vi "Read and Log Data.vi"(6 "Test No.":i32, 7 "Voltage Threshold":dbl=100.0, 8 "error in":errorcluster, 9 "Only Temperature":bool, 10 "Data":waveform(dbl)[](array[waveform]), 11 "tdms file":refnum<k34>) -> (0 "error out":errorcluster, 2 "Voltage Less Than Threshold":bool, 3 "tdms file out":refnum<k34>)   [LabVIEW 2015]
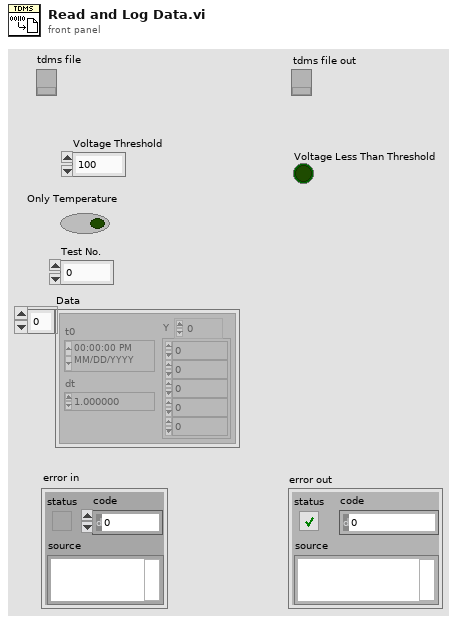
[diagram p1: front panel]
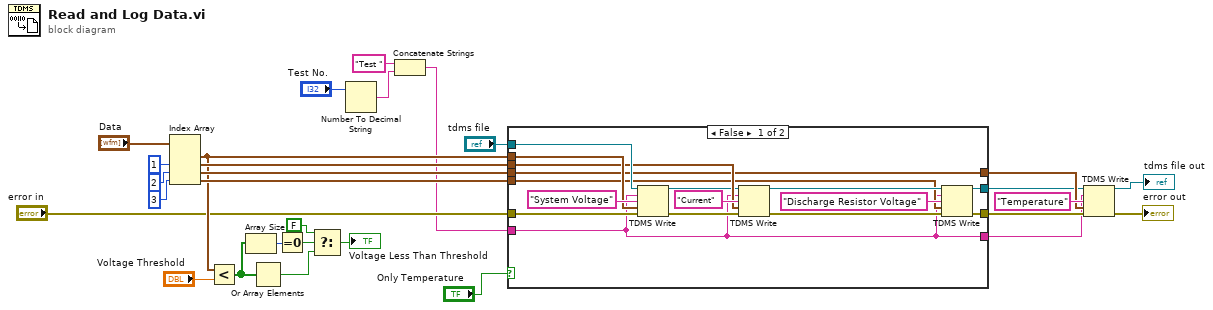
[diagram p0: block diagram]
diagram:
  n1 = Index Array(array="Data", index #2=1 ("index"), index #3=2 ("index"), index #4=3 ("index")) -> (element #1=w8:waveform(dbl), element #2=w24:waveform(dbl), element #3=w23:waveform(dbl), element #4=w19:waveform(dbl))  [unwired: 1 in]
  n2 = Less?(x=w8, y="Voltage Threshold") -> (x < y?=w12:bool[])
  n3 = Array Size(array=w12) -> (size(s)=w22:i32)
  n4 = Or Array Elements(Boolean array=w12) -> (logical OR=w11:bool)
  n5 = Equal To 0?(x=w22) -> (x = 0?=w21:bool)
  n6 = Select(t=FALSE, s=w21, f=w11) -> (s? t:f=→"Voltage Less Than Threshold":bool)
  n7 = Number To Decimal String(number="Test No.") -> (decimal integer string=w5:string)  [unwired: 1 in]
  n8 = Concatenate Strings("Test " ("string"), w5) -> (w3:string)
  n9 = case shown="False" "Only Temperature" {
    tunnel: "error in" -> [w44 w48]
    tunnel: w8 -> [w43 _]
    tunnel: "tdms file" -> [w42 w49]
    tunnel: w24 -> [w39 _]
    tunnel: w23 -> [w31 w47]
    tunnel: [w33 w48] -> w18
    tunnel: [w32 w49] -> w15
    tunnel: w19 -> [w34 _]
    tunnel: [w31 w47] -> w16
    tunnel: w3 -> [w30 w46]
    tunnel: [w30 w46] -> w2
    frame False {
      n10 = TDMS Write(0:w42, 5:w30, 7:"System Voltage" ("channel name(s) in (Untitled)"), 9:w43, 11:w44) -> (4:w38:refnum<k34>, 15:w41:errorcluster)  [unwired: 1 in, 2 out]
      n11 = TDMS Write(0:w38, 5:w30, 7:"Current" ("channel name(s) in (Untitled)"), 9:w39, 11:w41) -> (4:w35:refnum<k34>, 15:w37:errorcluster)  [unwired: 1 in, 2 out]
      n12 = TDMS Write(0:w35, 5:w30, 7:"Discharge Resistor Voltage" ("channel name(s) in (Untitled)"), 9:w34, 11:w37) -> (4:w32:refnum<k34>, 15:w33:errorcluster)  [unwired: 1 in, 2 out]
    }
    frame True {
    }
  }
  n13 = TDMS Write(0:w15, 5:w2, 7:"Temperature" ("channel name(s) in (Untitled)"), 9:w16, 11:w18) -> (4:→"tdms file out":refnum<k34>, 15:→"error out":errorcluster)  [unwired: 1 in, 2 out]
